vi "S8300E_ASKDisplayCard.vi"(3 "String":string) -> ()   [LabVIEW 2011]
doc: "This is an example of how to use the radio buttons control with the Value Changed event."
panel:
  out "Begin Time":u32
  in  "Pass Button":enum32{"No Selection", "Pass", "None"}(radio)=enum."Pass"
  out "NewVal":enum32{"No Selection", "NG", "None"}(ring)
  in  "NG Button":enum32{"No Selection", "NG", "None"}(radio)=enum."NG"
  # "顯卡目檢"
  # "2014-12-15"
  # "LCD Display 有顯示正常?"
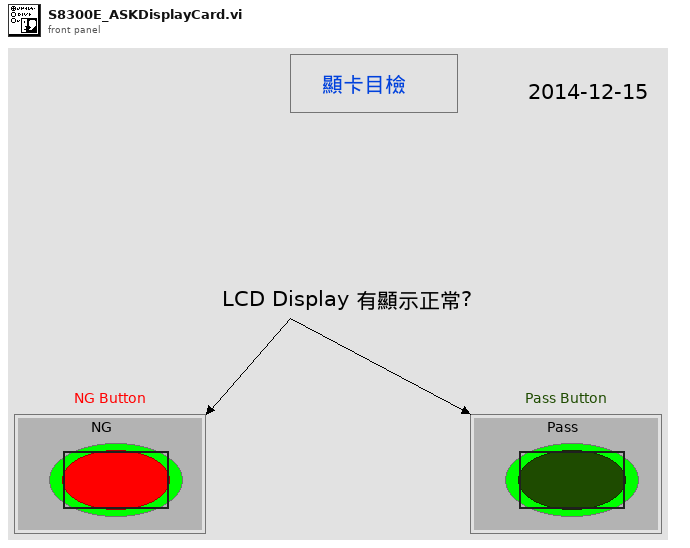
[diagram p1: front panel]
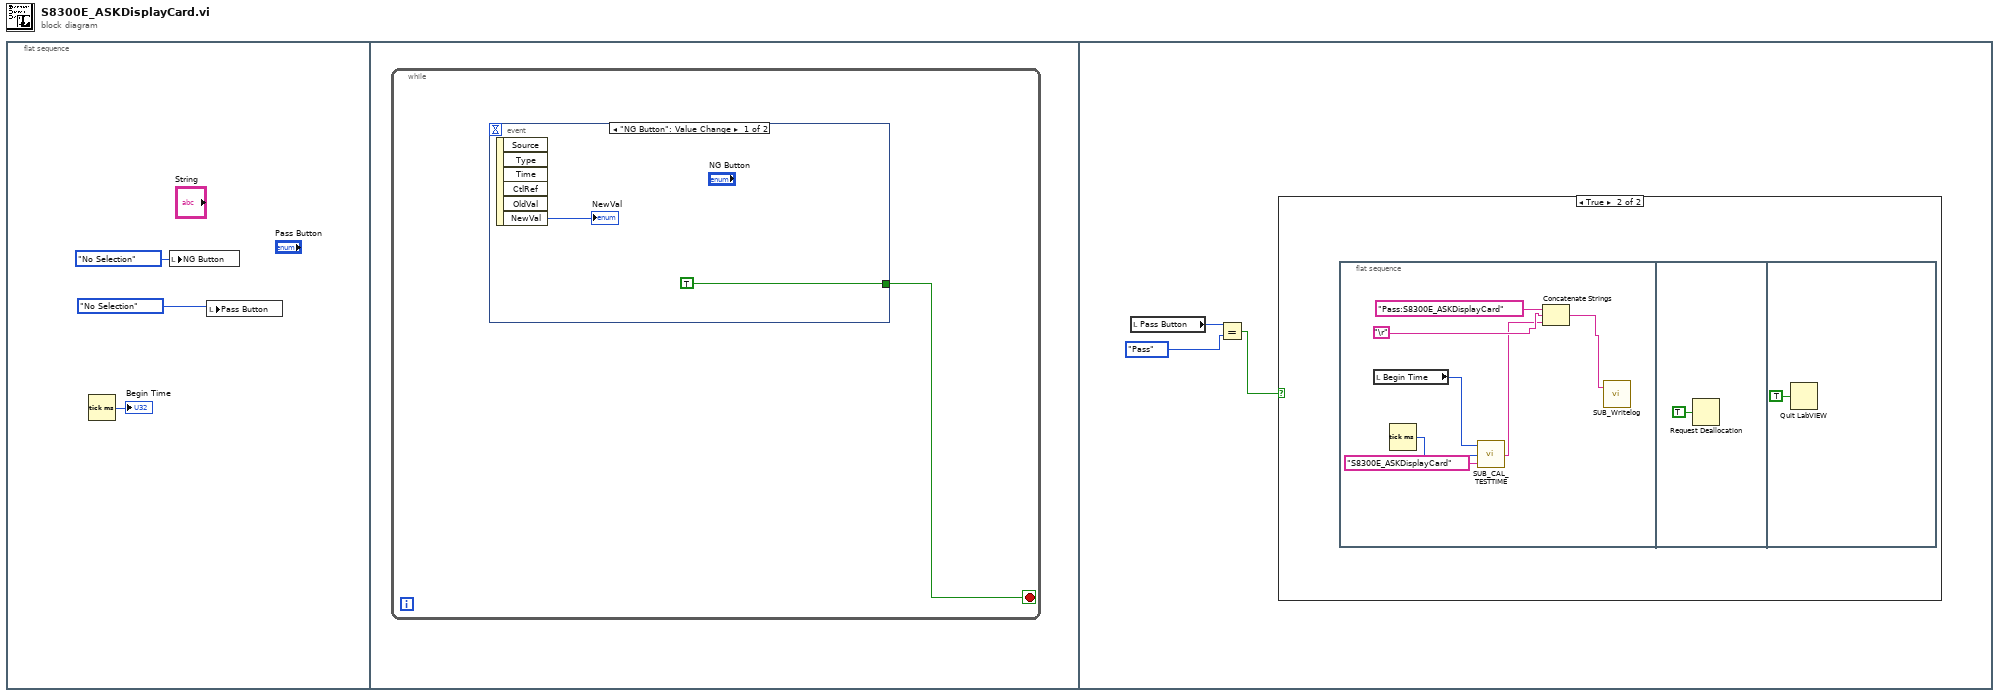
[diagram p0: block diagram]
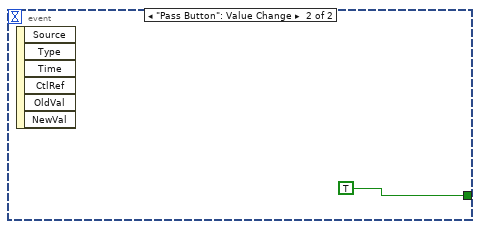
[diagram p2: hidden frame]
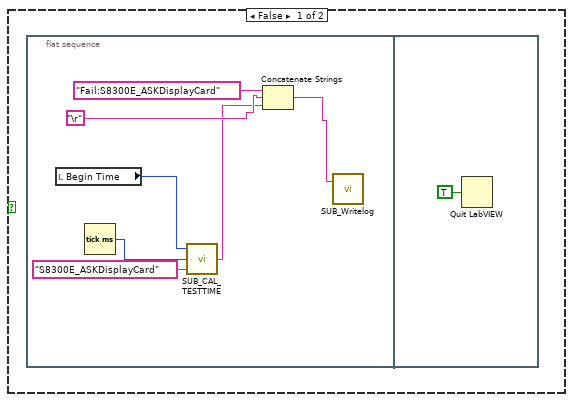
[diagram p3: hidden frame]
diagram:
  n1 = flat-sequence {
    frame #0 {
      n2 = Tick Count (ms)() -> (millisecond timer value=→"Begin Time":u32)
      n3 = local write "NG Button"(enum32{"No Selection", "NG", "None"}."No Selection" ("NG Button")) -> ()
      n4 = local write "Pass Button"(enum32{"No Selection", "Pass", "None"}."No Selection" ("Pass Button")) -> ()
    }
    frame #1 {
      n5 = while {
        stop <- w4 stop-if-true
        n6 = event shown="[0] \"NG Button\": Value Change" {
          selector: _ -> [_ _]
          dyn-events: _ -> [_ _]
          timeout: _ -> [_ _]
          tunnel: [TRUE TRUE] -> w4
          event "NG Button": Value Change {
            n7 = event-data() -> ("NewVal"=→"NewVal":enum32{"No Selection", "NG", "None"})  [unwired: 1 in, 5 out]
          }
          event "Pass Button": Value Change {
            n8 = event-data() -> ()  [unwired: 1 in, 6 out]
          }
        }
      }
    }
    frame #2 {
      n9 = local read "Pass Button"() -> (w10:enum32{"No Selection", "Pass", "None"})
      n10 = Equal?(x=w10, y=enum32{"No Selection", "Pass", "None"}."Pass") -> (x = y?=w8:bool)
      n11 = case shown="True" w8 {
        frame False {
          n12 = flat-sequence {
            frame #0 {
              n13 = local read "Begin Time"() -> (w11:u32)
              n14 = Tick Count (ms)() -> (millisecond timer value=w17:u32)
              n15 = call "SUB_CAL_TESTTIME.vi"("Test Item name"="S8300E_ASKDisplayCard", "Stop tick time"=w17, "Start tick time"=w11) -> ("Test Time output"=w13:string)  [unwired: 2 in]
              n16 = Concatenate Strings("Fail:S8300E_ASKDisplayCard" ("Pass/Fail"), "\r", w13) -> (w12:string)
              n17 = call "SUB_Writelog.vi"("Pass/Fail"=w12) -> ()  [unwired: 2 in]
            }
            frame #1 {
              n18 = Quit LabVIEW(quit? (T)=TRUE) -> ()
            }
          }
        }
        frame True {
          n19 = flat-sequence {
            frame #0 {
              n20 = local read "Begin Time"() -> (w19:u32)
              n21 = Tick Count (ms)() -> (millisecond timer value=w25:u32)
              n22 = call "SUB_CAL_TESTTIME.vi"("Test Item name"="S8300E_ASKDisplayCard", "Stop tick time"=w25, "Start tick time"=w19) -> ("Test Time output"=w21:string)  [unwired: 2 in]
              n23 = Concatenate Strings("Pass:S8300E_ASKDisplayCard" ("Pass/Fail"), "\r", w21) -> (w20:string)
              n24 = call "SUB_Writelog.vi"("Pass/Fail"=w20) -> ()  [unwired: 2 in]
            }
            frame #1 {
              n25 = Request Deallocation(TRUE ("flag")) -> ()
            }
            frame #2 {
              n26 = Quit LabVIEW(quit? (T)=TRUE) -> ()
            }
          }
        }
      }
    }
  }
